vi "Add PV (NT Enum (Reference)).vi"(5 "is read only? (F)":bool, 6 "initial timestamp":timestamp, 7 "PV name":string, 8 "error in (no error)":errorcluster, 10 "ref":refnum<vi>, 11 "Server in":refnum<class "Server.lvclass">) -> (0 "error out":errorcluster, 2 "ref out":refnum<vi>, 3 "Server out":refnum<class "Server.lvclass">, 4 "timestamp out":timestamp)   [LabVIEW 2020, in "PV Access.lvlib" / "PVA Server.lvlib" / "Server.lvclass"]
uses:
  Server.lvclass
  PV Data/NT Enum/NT Enum.lvclass
  C:/Users/eyw68381/source/repos/pvaccess-labview/labview/source/PV Data/NT Base/NT Base.lvclass
  Server.lvclass/Server.ctl
  Source/Source.lvclass
  PV Data/PV Data.lvlib
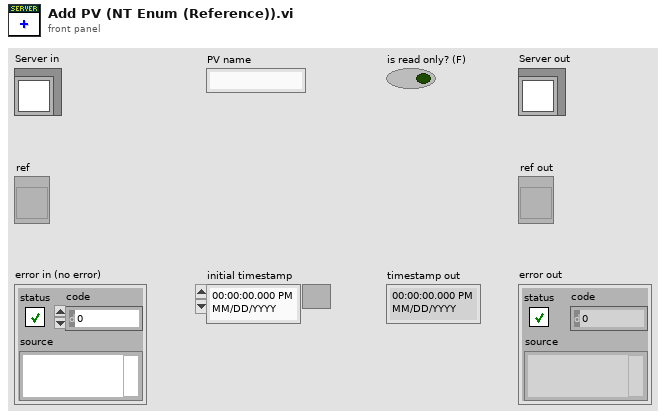
[diagram p1: front panel]
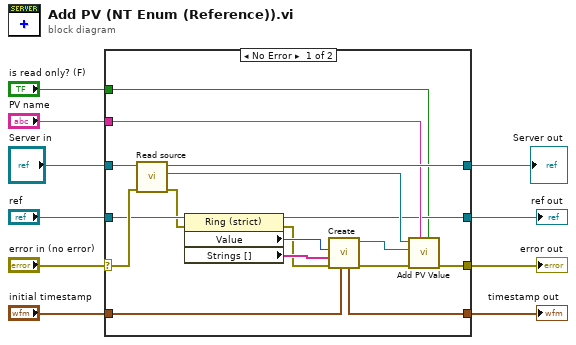
[diagram p0: block diagram]
diagram:
  n1 = case shown="No Error" "error in (no error)" {
    selector: "error in (no error)" -> [w23 w31]
    tunnel: [w22 w31] -> w9
    tunnel: [w26 w30] -> w7
    tunnel: "Server in" -> [w27 w30]
    tunnel: "PV name" -> [w24 _]
    tunnel: "initial timestamp" -> [w19 w29]
    tunnel: [w18 w29] -> w4
    tunnel: "ref" -> [w17 w28]
    tunnel: [w12 w28] -> w2
    tunnel: "is read only? (F)" -> [w11 _]
    frame No Error {
      n2 = call "Read source.vi"("error in (no error)"=w23, "Server in"=w27) -> ("error out"=w16:errorcluster, "Source"=w25:refnum<class "Source.lvclass">, "Server out"=w26:refnum<class "Server.lvclass">)  [unwired: 7 in]
      n3 = property class="Ring (strict)"(reference=w17, error in=w16) -> (reference out=w12:refnum<vi>, error out=w13:errorcluster, "Value"=w15:u16, "Strings []"=w14:string[])
      n4 = call-poly "Create.vi"("initial timestamp"=w19, "error in (no error)"=w13, "choices"=w14, "initial index"=w15) -> ("error out"=w21:errorcluster, "NT Enum out"=w20:refnum<class "NT Enum.lvclass">, "timestamp out"=w18:timestamp)  [unwired: 3 in, 2 out]
      n5 = call "Add PV Value.vi"("is read only? (F)"=w11, "PV name"=w24, "error in"=w21, "NT Base in"=w20, "Source in"=w25) -> ("error out"=w22:errorcluster)  [unwired: 4 in, 2 out]
    }
    frame Error {
    }
  }
  "error out" <- w9
  "Server out" <- w7
  "timestamp out" <- w4
  "ref out" <- w2
